vi "mtg - module.vi"(7 "action":T3=enum."update data", 8 "error in (no error)":errorcluster, 9 "graph selection":T2(ring), 10 "value references":refnum<vi>[](array[refnum]), 11 "chart in":refnum<vi>) -> (0 "error out":errorcluster, 1 "1 hr History Data":dbl[][](array[numeric]), 2 "date time info":T1, 3 "chart out":refnum<vi>)   [LabVIEW 2025]
uses:
  mtg - action.ctl
panel:
  in  "pre-delay (1500 ms)":u32=1500
  out "store 1 s":dbl[][](graph)
  out "store 120 s":dbl[][](graph)
  out "store 60 s":dbl[][](graph)
  out "store 30 s":dbl[][](graph)
  out "store 5 s":dbl[][](graph)
  # "data storage"
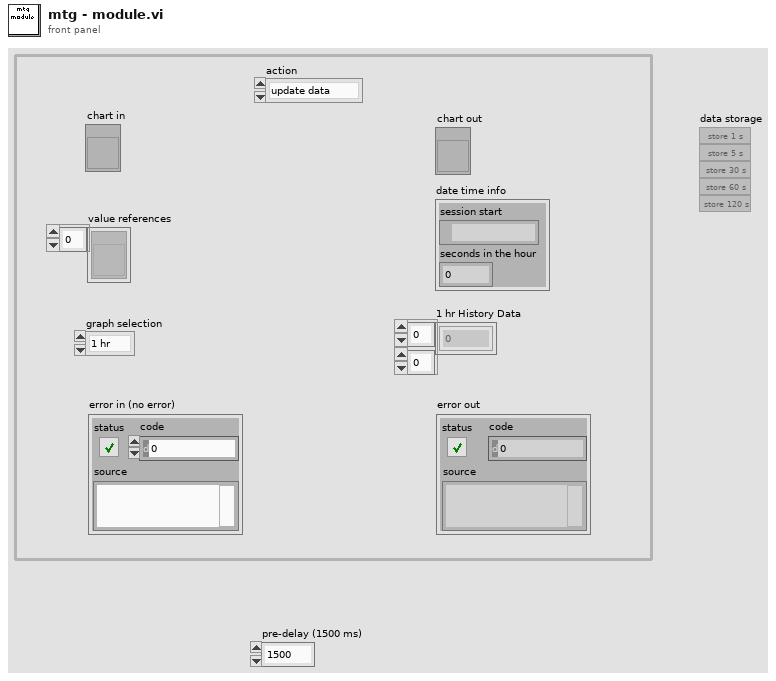
[diagram p1: front panel]
types:
  T1 = cluster{"session start":path, "seconds in the hour":i32}
  T2 = enum16{"1 hr", "5 hr", "30 hr", "60 hr", "120 hr", "1 hr (from file)"}
  T3 = typedef "mtg - action.ctl" = enum16{"init", "update data", "change timescale", "get data for file", "get final data for file", "set data from file"}
  T4 = cluster{"created path":path, "seconds into the hour":i32}
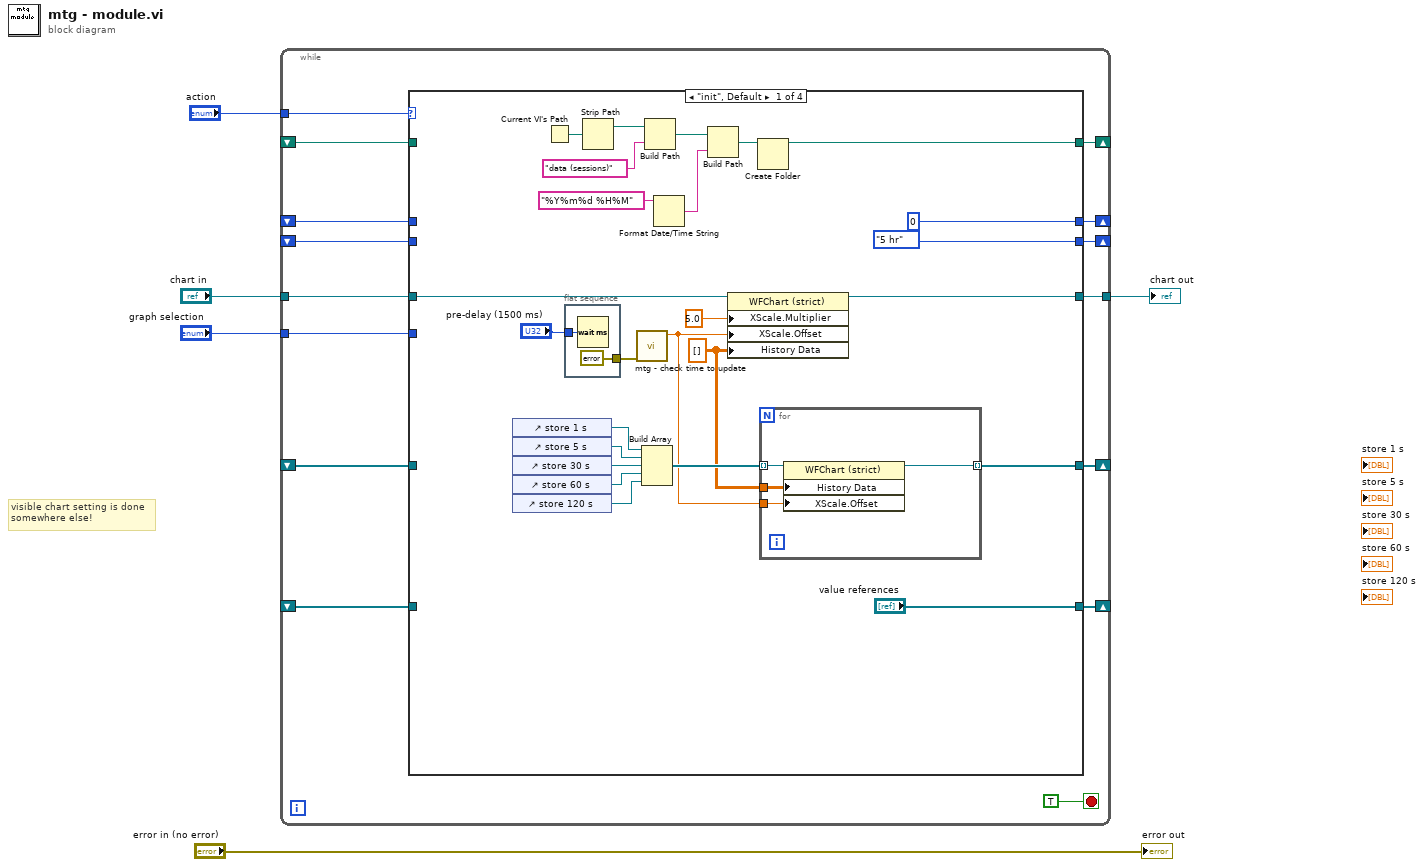
[diagram p0: block diagram]
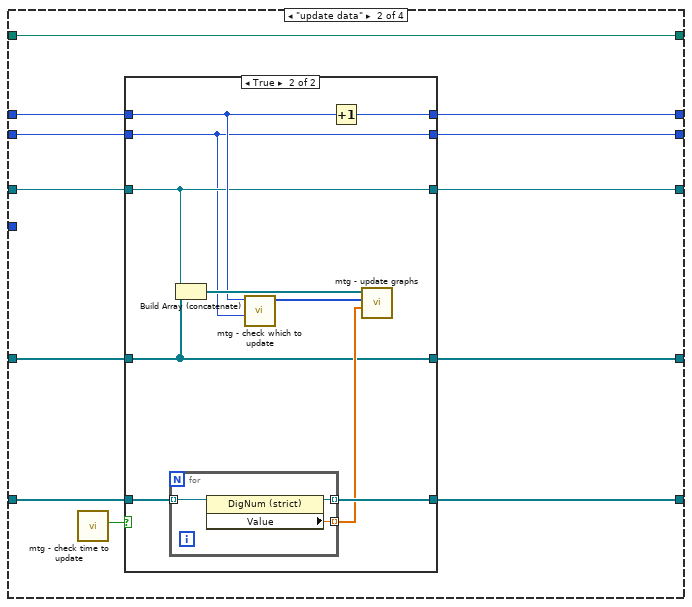
[diagram p2: hidden frame]
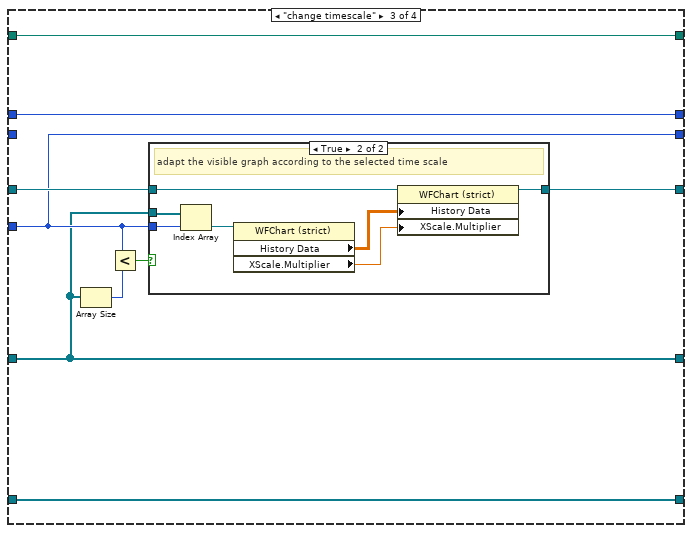
[diagram p4: hidden frame]
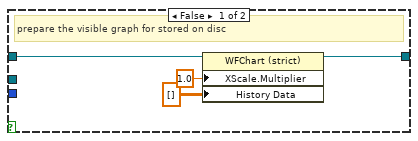
[diagram p5: hidden frame]
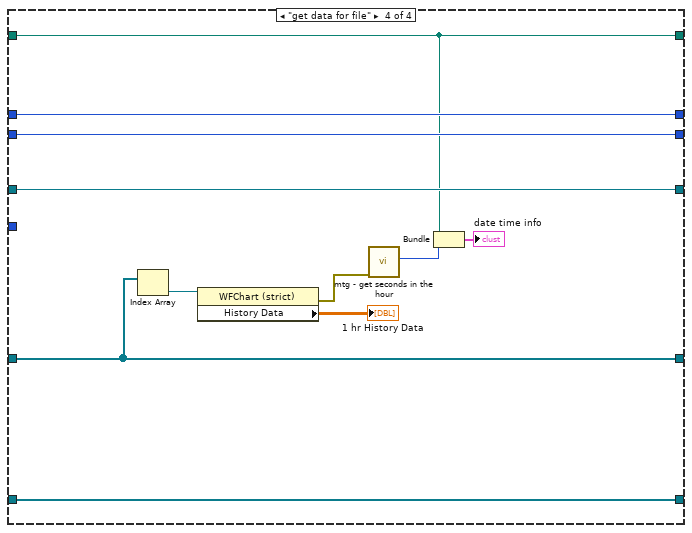
[diagram p6: hidden frame]
diagram:
  # "visible chart setting is done\nsomewhere else!"
  n1 = while {
    tunnel: "action" -> [w19]
    tunnel: "chart in" -> [w18]
    tunnel: [w17] -> w3
    shift-right: [w16] -> _
    shift-left: _ -> [w15]
    shift-right: [w14] -> _
    shift-left: _ -> [w13]
    shift-right: [w8] -> _
    shift-left: _ -> [w12]
    tunnel: "graph selection" -> [w11]
    shift-right: [w10] -> _
    shift-left: _ -> [w9]
    shift-right: [w7] -> _
    shift-left: _ -> [w6]
    stop <- TRUE stop-if-true
    n2 = case shown="\"init\", Default" w19 {
      tunnel: w18 -> [w35 w60 w90 w110]
      tunnel: [w34 w56 w87 w110] -> w17
      tunnel: [w31 w55 w85 w108] -> w16
      tunnel: w15 -> [_ w59 w85 w108]
      tunnel: ["value references" w62 w89 w109] -> w14
      tunnel: w13 -> [_ w63 w89 w109]
      tunnel: [0 w53 w88 w112] -> w8
      tunnel: w12 -> [_ w61 w88 w112]
      tunnel: w11 -> [_ _ w86 _]
      tunnel: [T2."5 hr" ("graph selection") w57 w86 w111] -> w10
      tunnel: w9 -> [_ w58 _ w111]
      tunnel: [w21 w52 w82 w104] -> w7
      tunnel: w6 -> [_ w52 w82 w104]
      frame "init", Default {
        w30 = dbl[][] [] ("History Data")
        n3 = control-ref of="store 1 s"() -> (w41:refnum<vi>)
        n4 = control-ref of="store 5 s"() -> (w42:refnum<vi>)
        n5 = control-ref of="store 30 s"() -> (w43:refnum<vi>)
        n6 = control-ref of="store 60 s"() -> (w44:refnum<vi>)
        n7 = control-ref of="store 120 s"() -> (w45:refnum<vi>)
        n8 = Current VI's Path() -> (path=w27:path)
        n9 = flat-sequence {
          tunnel: "pre-delay (1500 ms)" -> [w51]
          tunnel: [errorcluster {"status"=FALSE, "code"=0, "source"=""} ("error constant")] -> w36
          frame #0 {
            n10 = Wait (ms)(milliseconds to wait=w51) -> ()  [unwired: 1 out]
          }
        }
        n11 = Strip Path(path=w27) -> (stripped path=w26:path)  [unwired: 1 out]
        n12 = call "mtg - check time to update.vi"("error in (no error)"=w36) -> ("xscale offset"=w29:dbl)  [unwired: 8 in, 2 out]
        n13 = Build Array(w41, w42, w43, w44, w45) -> (w32:refnum<vi>[])
        n14 = Build Path(base path=w26, name or relative path="data (sessions)" ("time format string (%c)")) -> (appended path=w24:path)
        n15 = Format Date/Time String(time format string (%c)="%Y%m%d %H%M") -> (date/time string=w23:string)  [unwired: 2 in]
        n16 = Build Path(base path=w24, name or relative path=w23) -> (appended path=w22:path)
        n17 = property class="WFChart (strict)"(reference=w35, "XScale.Multiplier"=5.0 ("X Scale.Offset and Multiplier:Multiplier"), "XScale.Offset"=w29, "History Data"=w30) -> (reference out=w34:refnum<vi>)  [unwired: 1 in, 1 out]
        n18 = Create Folder(path (use dialog)=w22) -> (created path=w21:path)  [unwired: 2 in, 2 out]
        n19 = for {
          tunnel: w32 -> [w49] mode=indexing
          tunnel: [w48] -> w31 mode=indexing
          tunnel: w30 -> [w47]
          tunnel: w29 -> [w46]
          n20 = property class="WFChart (strict)"(reference=w49, "History Data"=w47, "XScale.Offset"=w46) -> (reference out=w48:refnum<vi>)  [unwired: 1 in, 1 out]
        }
      }
      frame "update data" {
        n21 = call "mtg - check time to update.vi"() -> ("get reading"=w54:bool)  [unwired: 9 in, 2 out]
        n22 = case shown="True" w54 {
          tunnel: w63 -> [w65 w78]
          tunnel: [w65 w77] -> w62
          tunnel: w61 -> [w64 w73]
          tunnel: w60 -> [w67 w71]
          tunnel: w59 -> [w66 w70]
          tunnel: [w64 w72] -> w53
          tunnel: w58 -> [w68 w69]
          tunnel: [w68 w69] -> w57
          tunnel: [w67 w71] -> w56
          tunnel: [w66 w70] -> w55
          frame False {
          }
          frame True {
            n23 = for {
              tunnel: w78 -> [w81] mode=indexing
              tunnel: [w80] -> w77 mode=indexing
              tunnel: [w79] -> w74 mode=indexing
              n24 = property class="DigNum (strict)"(reference=w81) -> (reference out=w80:refnum<vi>, "Value"=w79:dbl)  [unwired: 1 in, 1 out]
            }
            n25 = Build Array (concatenate)(w71, w70) -> (w75:refnum<vi>[])
            n26 = call "mtg - check which to update.vi"("graph selection"=w69, "iteration index (s)"=w73) -> ("update list (10...)"=w76:i32[])  [unwired: 9 in]
            n27 = Increment(x=w73) -> (x+1=w72:i32)
            n28 = call "mtg - update graphs.vi"("new data"=w74, "update list (10...)"=w76, "chart refs in"=w75) -> ()  [unwired: 7 in, 2 out]
          }
        }
      }
      frame "change timescale" {
        n29 = Array Size(array=w85) -> (size(s)=w84:i32)
        n30 = Less?(x=w86, y=w84) -> (x < y?=w83:bool)
        n31 = case shown="True" w83 {
          tunnel: w90 -> [w94 w101]
          tunnel: [w93 w100] -> w87
          tunnel: w86 -> [_ w96]
          tunnel: w85 -> [_ w95]
          frame False {
            # "prepare the visible graph for stored on disc"
            n32 = property class="WFChart (strict)"(reference=w94, "XScale.Multiplier"=1.0 ("X Scale.Offset and Multiplier:Multiplier"), "History Data"=dbl[][] []) -> (reference out=w93:refnum<vi>)  [unwired: 1 in, 1 out]
          }
          frame True {
            # "adapt the visible graph according to the selected time scale"
            n33 = Index Array(array=w95, index=w96) -> (element=w99:refnum<vi>)
            n34 = property class="WFChart (strict)"(reference=w99) -> ("History Data"=w98:dbl[][], "XScale.Multiplier"=w97:dbl)  [unwired: 1 in, 2 out]
            n35 = property class="WFChart (strict)"(reference=w101, "History Data"=w98, "XScale.Multiplier"=w97) -> (reference out=w100:refnum<vi>)  [unwired: 1 in, 1 out]
          }
        }
      }
      frame "get data for file" {
        n36 = Index Array(array=w108) -> (element=w107:refnum<vi>)  [unwired: 1 in]
        n37 = property class="WFChart (strict)"(reference=w107) -> (error out=w105:errorcluster, "History Data"=→"1 hr History Data":dbl[][])  [unwired: 1 in, 1 out]
        n38 = call "mtg - get seconds in the hour.vi"("error in (no error)"=w105) -> ("seconds into the hour"=w103:i32)  [unwired: 10 in]
        n39 = Bundle("created path"=w104, "seconds into the hour"=w103) -> (→"date time info":T4)  [unwired: 1 in]
      }
    }
  }
  "chart out" <- w3
  "error out" <- "error in (no error)"
